vi "SaveData.vi"(0 "object in":refnum<class "TDMSLogger.lvclass">, 1 "Elapsed Time":dbl, 2 "ChannelsWFIn":waveform(dbl)[](array[waveform]), 3 "AmplitudeAndVoltageSettings":T4, 4 "MeTecData":T3={"meTEC_CH2_Temperature Stability"=1, "meTEC_CH2_Act. Output Current [A]"=0.0, "meTEC_CH2_Act. Output Voltage [V]"=0.0, "meTEC_CH2_Object Temperature [°C]"=0.0, "meTEC_CH2_Sink Temperature [°C]"=0.0, "meTEC_CH1_Error Parameter"=0, "meTEC_CH1_Error Instance"=0, "meTEC_CH1_Error No."=0, "meTEC_CH1_Device Status"=1, "meTEC_CH1_Temperature Stability"=1, "meTEC_CH1_Act. Output Current [A]"=0.0, "meTEC_CH1_Act. Output Voltage [V]"=0.0, "meTEC_CH1_Object Temperature [°C]"=0.0, "meTEC_CH1_Sink Temperature [°C]"=0.0} {"meTEC_CH1_Sink Temperature [°C]" format="%.3f"; "meTEC_CH1_Object Temperature [°C]" format="%.3f"; "meTEC_CH1_Act. Output Voltage [V]" format="%.3f"; "meTEC_CH1_Act. Output Current [A]" format="%.3f"; "meTEC_CH1_Temperature Stability" items=["Temperature regulation is not active", "Is not stable", "Is stable"]; "meTEC_CH1_Device Status" items=["Initializing", "Ready", "Run", "Error", "Bootloader", "Reset in Progress"]; "meTEC_CH2_Sink Temperature [°C]" format="%.3f"; "meTEC_CH2_Object Temperature [°C]" format="%.3f"; "meTEC_CH2_Act. Output Voltage [V]" format="%.3f"; "meTEC_CH2_Act. Output Current [A]" format="%.3f"; "meTEC_CH2_Temperature Stability" items=["Temperature regulation is not active", "Is not stable", "Is stable"]}, 5 "error in (no error)":errorcluster, 6 "AGTemp":dbl, 7 "SetPower":dbl, 8 "MCCTempdata":dbl[](array[numeric]), 9 "MeasuredPower":dbl, 11 "AmplitudeOk":bool, 13 "WfgEnabled":cluster{"Ch1":bool, "Ch2":bool}) -> (14 "object out":refnum<class "TDMSLogger.lvclass">, 19 "error out":errorcluster)   [LabVIEW 2019, in "TDMSLogger.lvclass"]
uses:
  TDMSLogger.lvclass
  TEC LabVIEW Control Software v0.14/Source/LV Source/[meerstetter engineering TE Cooling]/TypeDefs/meTEC_ID 1200_Temperature is Stable.ctl
  TEC LabVIEW Control Software v0.14/Source/LV Source/[meerstetter engineering TE Cooling]/TypeDefs/meTEC_ID 104_Device Status.ctl
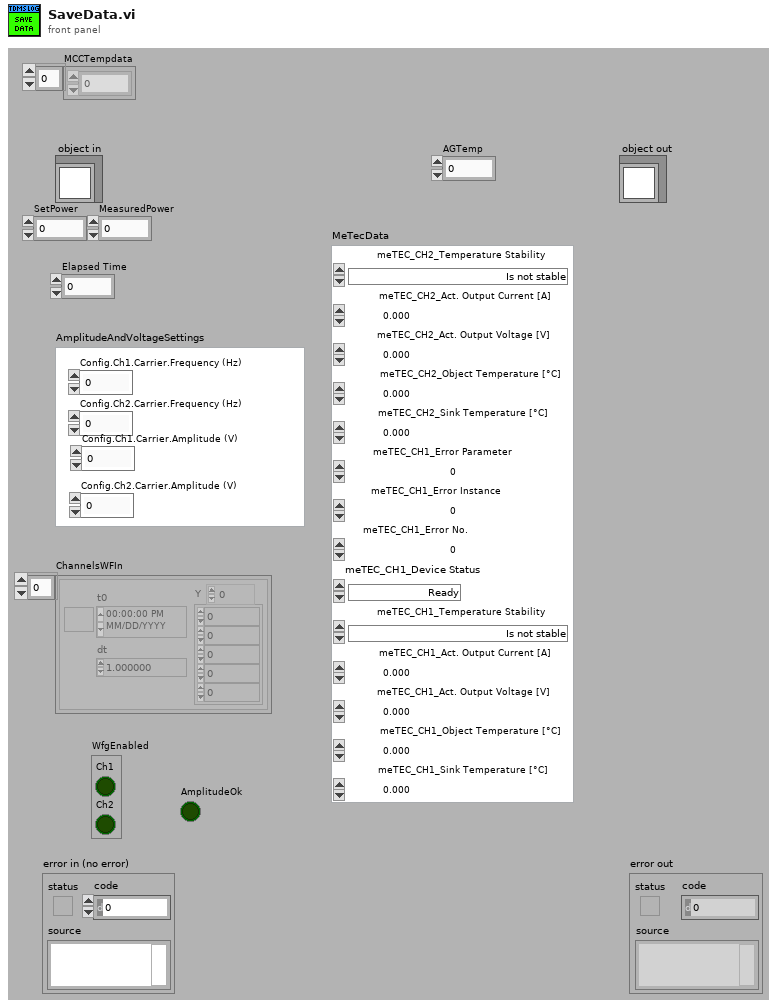
[diagram p1: front panel]
types:
  T1 = typedef "meTEC_ID 1200_Temperature is Stable.ctl" = i32
  T2 = typedef "meTEC_ID 104_Device Status.ctl" = i32
  T3 = cluster{"meTEC_CH2_Temperature Stability":T1, "meTEC_CH2_Act. Output Current [A]":dbl, "meTEC_CH2_Act. Output Voltage [V]":dbl, "meTEC_CH2_Object Temperature [°C]":dbl, "meTEC_CH2_Sink Temperature [°C]":dbl, "meTEC_CH1_Error Parameter":i32, "meTEC_CH1_Error Instance":i32, "meTEC_CH1_Error No.":i32, "meTEC_CH1_Device Status":T2, "meTEC_CH1_Temperature Stability":T1, "meTEC_CH1_Act. Output Current [A]":dbl, "meTEC_CH1_Act. Output Voltage [V]":dbl, "meTEC_CH1_Object Temperature [°C]":dbl, "meTEC_CH1_Sink Temperature [°C]":dbl}
  T4 = cluster{"Config.Ch1.Carrier.Frequency (Hz)":dbl, "Config.Ch2.Carrier.Frequency (Hz)":dbl, "Config.Ch1.Carrier.Amplitude (V)":dbl, "Config.Ch2.Carrier.Amplitude (V)":dbl}
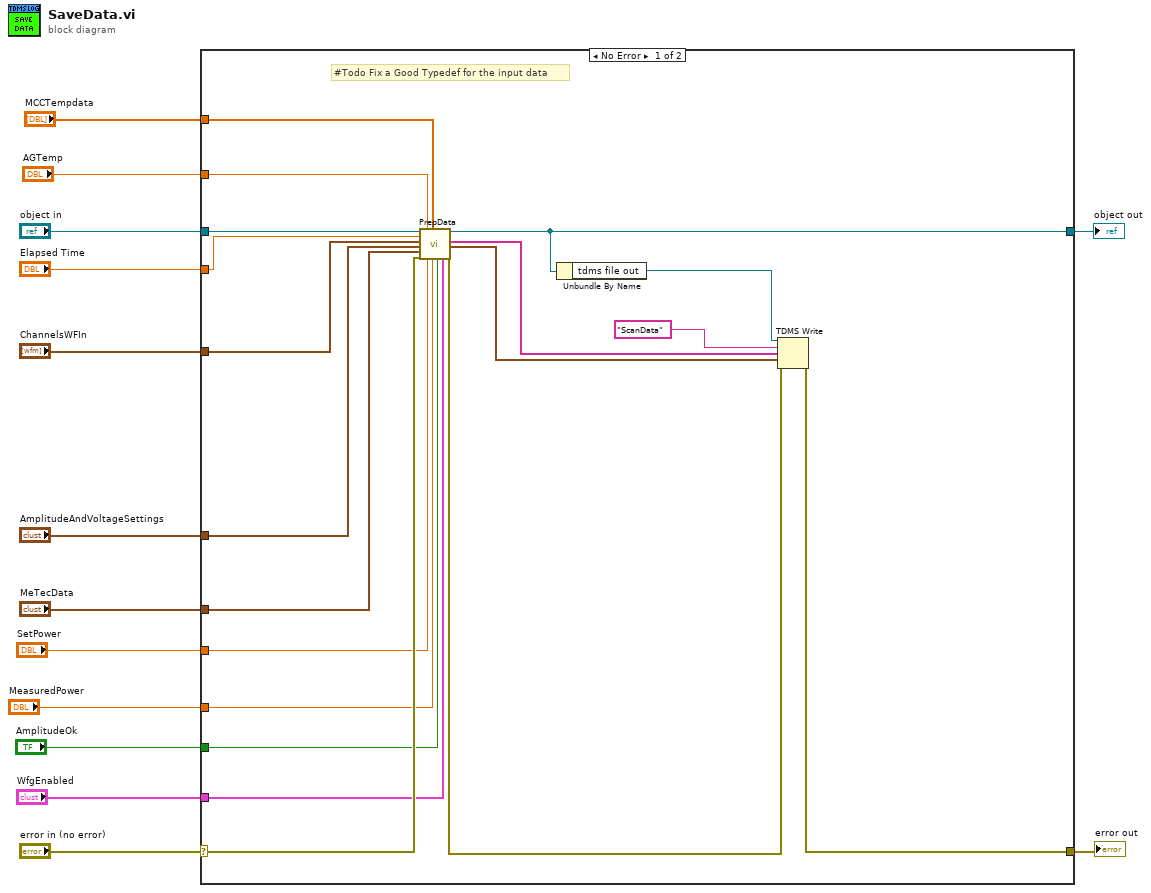
[diagram p0: block diagram]
diagram:
  n1 = case shown="No Error" "error in (no error)" {
    selector: "error in (no error)" -> [w26 w35]
    tunnel: [w30 w35] -> w13
    tunnel: [w24 w34] -> w11
    tunnel: "object in" -> [w29 w34]
    tunnel: "AmplitudeAndVoltageSettings" -> [w33 _]
    tunnel: "ChannelsWFIn" -> [w31 _]
    tunnel: "Elapsed Time" -> [w28 _]
    tunnel: "MeTecData" -> [w27 _]
    tunnel: "SetPower" -> [w20 _]
    tunnel: "MeasuredPower" -> [w19 _]
    tunnel: "AmplitudeOk" -> [w18 _]
    tunnel: "WfgEnabled" -> [w17 _]
    tunnel: "AGTemp" -> [w16 _]
    tunnel: "MCCTempdata" -> [w15 _]
    frame No Error {
      # "#Todo Fix a Good Typedef for the input data"
      n2 = call-dynamic "PrepData.vi"("object in"=w29, "Elapsed Time"=w28, "ChannelsWFIn"=w31, "AmplitudeAndVoltageSettings"=w33, "MeTecData"=w27, "error in (no error)"=w26, "AGTemp"=w16, "SetPower"=w20, "MCC TempData"=w15, "MeasuredPower"=w19, "AmplitudeOk"=w18, "WfgEnabled"=w17) -> ("object out"=w24:refnum<class "TDMSLogger.lvclass">, "Channel Names"=w23:string[], "Channels(WF)"=w22:waveform(dbl)[], "error out"=w25:errorcluster)  [unwired: 4 in]
      n3 = Unbundle By Name(w24) -> ("tdms file out"=w21:refnum<k34>)
      n4 = TDMS Write(0:w21, 5:"ScanData" ("group name in (Untitled)"), 7:w23, 9:w22, 11:w25) -> (15:w30:errorcluster)  [unwired: 1 in, 3 out]
    }
    frame Error {
    }
  }
  "error out" <- w13
  "object out" <- w11
